vi "(SubVI)SAI_PANEL_CODIGO.vi"(0 "Modbus Master in":refnum<class "Modbus Master.lvclass">, 5 "error in (no error)":errorcluster) -> (6 "bypass(F), line (T)":bool, 7 "salida Vs":dbl, 8 "Tin":u16, 9 "corriente S":dbl format="%.2f", 10 "Sin":u16, 11 "salida Vr":dbl, 12 "Work mode":string, 13 "corriente R":dbl format="%.2f", 14 "Modbus Master out":refnum<class "Modbus Master.lvclass">, 15 "Rin":u16, 16 "corrinte T":dbl format="%.2f", 17 "Porcentaje P":dbl, 18 "salida Vt":dbl, 19 "error out":errorcluster)   [LabVIEW 2024, in "SALICRU_MODBUS.lvlib"]
uses:
  <vilib>/Modbus/master/Modbus Master.lvclass
  SALICRU_MODBUS.lvlib
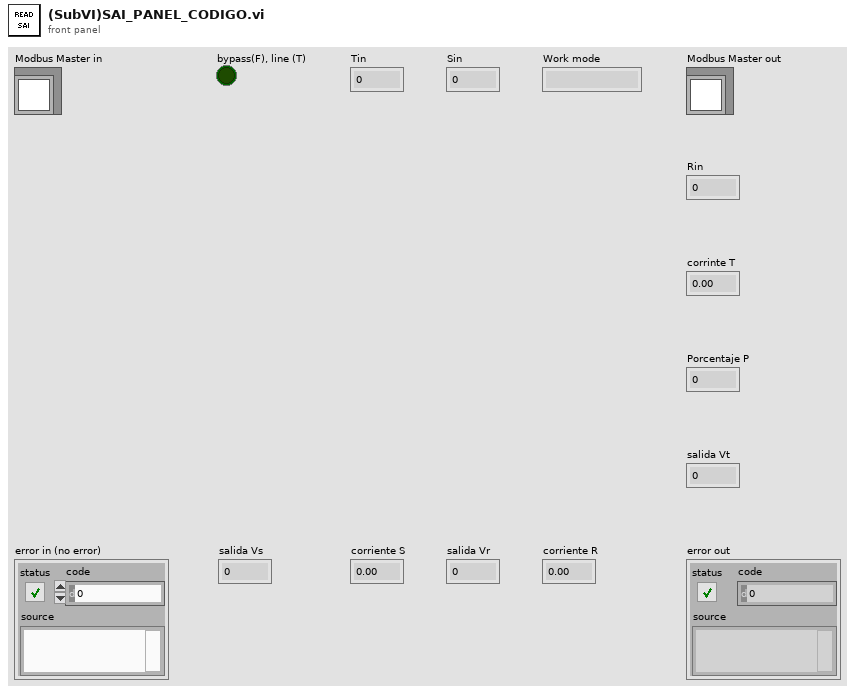
[diagram p1: front panel]
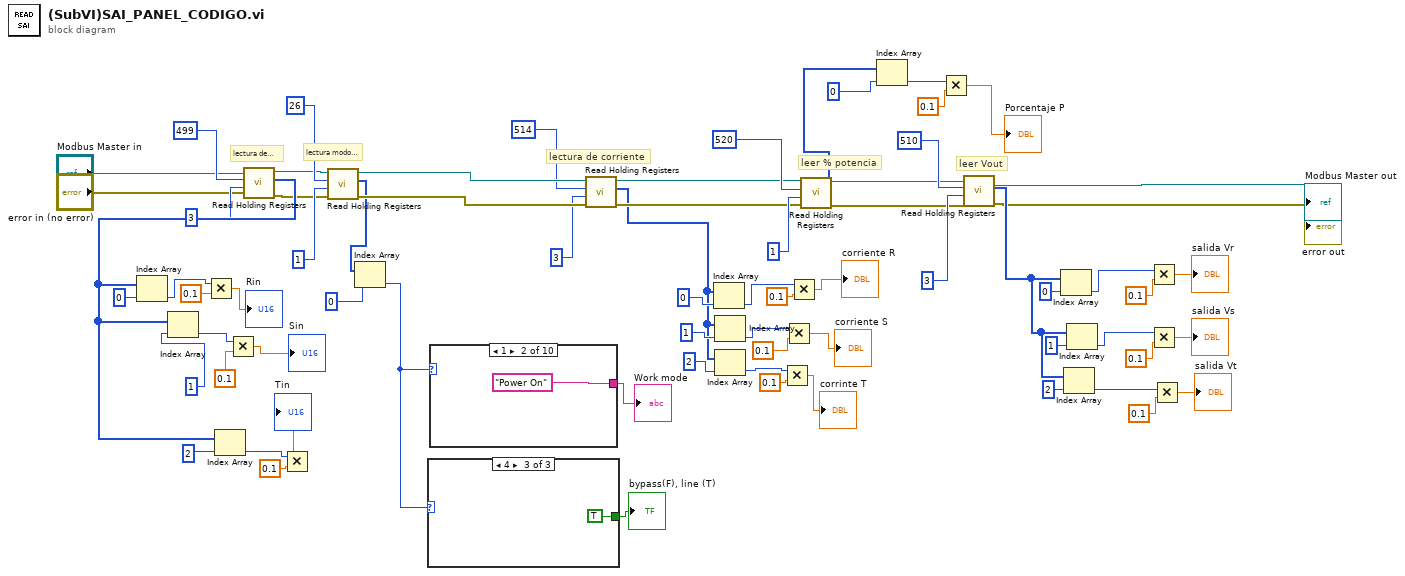
[diagram p0: block diagram]
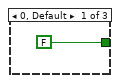
[diagram p2: hidden frame]
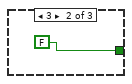
[diagram p3: hidden frame]
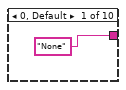
[diagram p4: hidden frame]
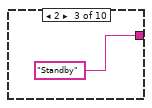
[diagram p5: hidden frame]
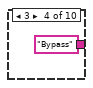
[diagram p6: hidden frame]
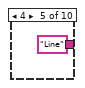
[diagram p7: hidden frame]
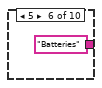
[diagram p8: hidden frame]
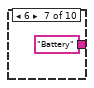
[diagram p9: hidden frame]
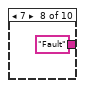
[diagram p10: hidden frame]
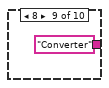
[diagram p11: hidden frame]
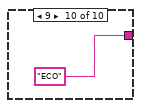
[diagram p12: hidden frame]
diagram:
  # "leer Vout"
  # "leer % potencia"
  # "lectura de corriente"
  # "lectura modos de trabajo"
  # "lectura de tensiones de entrada"
  n1 = call-dynamic "Read Holding Registers.vi"("error in (no error)"="error in (no error)", "number of holding registers"=u16 3, "starting address"=u16 499, "Modbus master in"="Modbus Master in") -> ("error out"=w6:errorcluster, "register values"=w15:u16[], "Modbus master out"=w5:refnum<class "Modbus Master.lvclass">)  [unwired: 5 in]
  n2 = Index Array(array=w15, index=0) -> (element=w22:u16)
  n3 = Index Array(array=w15, index=1) -> (element=w24:u16)
  n4 = Multiply(x=w22, y=0.1) -> (x*y=→"Rin":dbl)
  n5 = Index Array(array=w15, index=2) -> (element=w28:u16)
  n6 = Multiply(x=w24, y=0.1) -> (x*y=→"Sin":dbl)
  n7 = Multiply(x=w28, y=0.1) -> (x*y=→"Tin":dbl)
  n8 = call-dynamic "Read Holding Registers.vi"("error in (no error)"=w6, "number of holding registers"=u16 1, "starting address"=u16 26, "Modbus master in"=w5) -> ("error out"=w58:errorcluster, "register values"=w8:u16[], "Modbus master out"=w57:refnum<class "Modbus Master.lvclass">)  [unwired: 5 in]
  n9 = Index Array(array=w8, index=0) -> (element=w11:u16)
  n10 = case shown="4" w11 {
    tunnel: [FALSE FALSE TRUE] -> w12
    frame 0, Default {
    }
    frame 3 {
    }
    frame 4 {
    }
  }
  "bypass(F), line (T)" <- w12
  n11 = case shown="1" w11 {
    tunnel: ["None" "Power On" "Standby" "Bypass" "Line" "Batteries" "Battery" "Fault" "Converter" "ECO"] -> w10
    frame 0, Default {
    }
    frame 1 {
    }
    frame 2 {
    }
    frame 3 {
    }
    frame 4 {
    }
    frame 5 {
    }
    frame 6 {
    }
    frame 7 {
    }
    frame 8 {
    }
    frame 9 {
    }
  }
  "Work mode" <- w10
  n12 = call-dynamic "Read Holding Registers.vi"("error in (no error)"=w58, "number of holding registers"=u16 3, "starting address"=u16 514, "Modbus master in"=w57) -> ("error out"=w43:errorcluster, "register values"=w19:u16[], "Modbus master out"=w42:refnum<class "Modbus Master.lvclass">)  [unwired: 5 in]
  n13 = Index Array(array=w19, index=0) -> (element=w31:u16)
  n14 = Index Array(array=w19, index=1) -> (element=w34:u16)
  n15 = Index Array(array=w19, index=2) -> (element=w37:u16)
  n16 = Multiply(x=w37, y=0.1) -> (x*y=→"corrinte T":dbl)
  n17 = Multiply(x=w34, y=0.1) -> (x*y=→"corriente S":dbl)
  n18 = Multiply(x=w31, y=0.1) -> (x*y=→"corriente R":dbl)
  n19 = call-dynamic "Read Holding Registers.vi"("error in (no error)"=w43, "number of holding registers"=u16 1, "starting address"=u16 520, "Modbus master in"=w42) -> ("error out"=w52:errorcluster, "register values"=w46:u16[], "Modbus master out"=w51:refnum<class "Modbus Master.lvclass">)  [unwired: 5 in]
  n20 = Index Array(array=w46, index=0) -> (element=w49:u16)
  n21 = Multiply(x=w49, y=0.1) -> (x*y=→"Porcentaje P":dbl)
  n22 = call-dynamic "Read Holding Registers.vi"("error in (no error)"=w52, "number of holding registers"=u16 3, "starting address"=u16 510, "Modbus master in"=w51) -> ("error out"=→"error out":errorcluster, "register values"=w59:u16[], "Modbus master out"=→"Modbus Master out":refnum<class "Modbus Master.lvclass">)  [unwired: 5 in]
  n23 = Index Array(array=w59, index=0) -> (element=w66:u16)
  n24 = Index Array(array=w59, index=2) -> (element=w68:u16)
  n25 = Index Array(array=w59, index=1) -> (element=w67:u16)
  n26 = Multiply(x=w66, y=0.1) -> (x*y=→"salida Vr":dbl)
  n27 = Multiply(x=w67, y=0.1) -> (x*y=→"salida Vs":dbl)
  n28 = Multiply(x=w68, y=0.1) -> (x*y=→"salida Vt":dbl)
